vi "产品工艺设定.vi"() -> ()   [LabVIEW 2020]
panel:
  out "ALL_DEVICE":string[](array[string])
  in  "确定":bool
  in  "产品型号":u16(ring) items=[""=0, "R128"=1, "R527"=4, "R538"=5, "R92A"=3]
  in  "产品工艺":string(tree)
  in  "工位名称":i32(listbox)
  out "data":string[][](array[string])
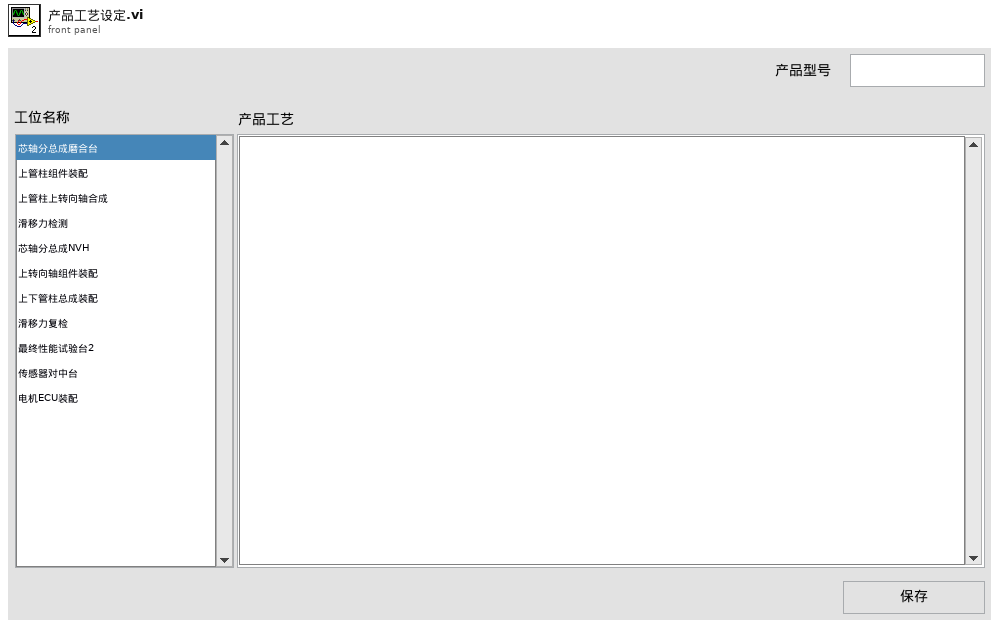
[diagram p1: front panel]
types:
  T1 = cluster{"data name":string, "drag data":variant}[]
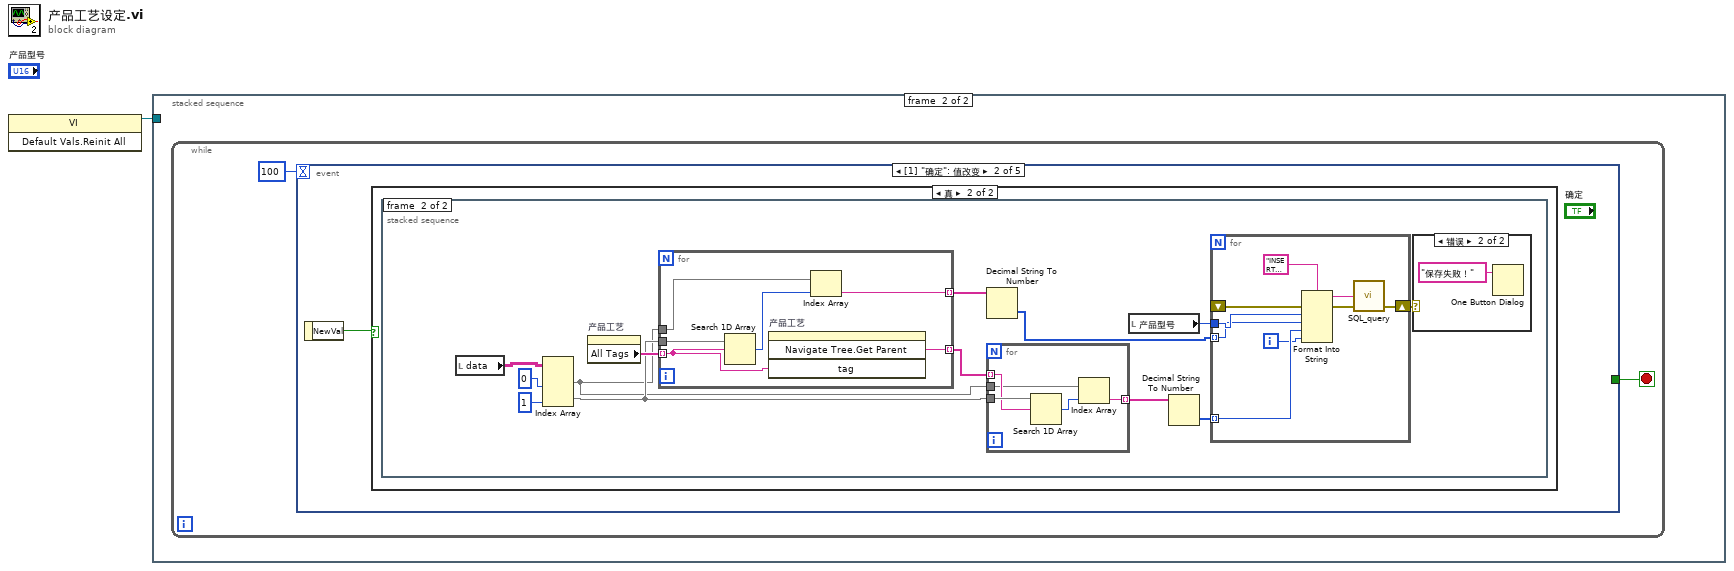
[diagram p0: block diagram]
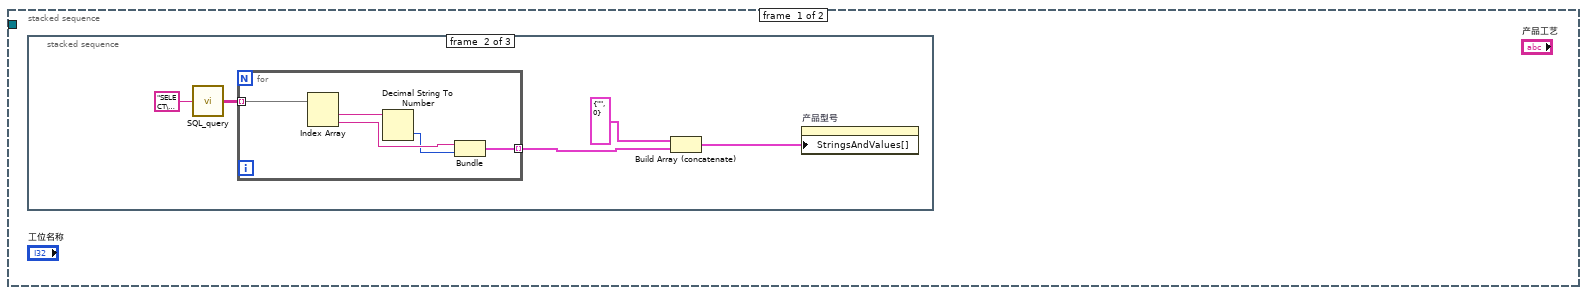
[diagram p2: hidden frame]
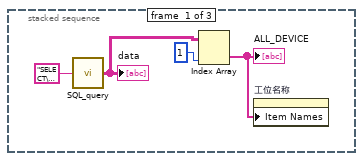
[diagram p3: hidden frame]
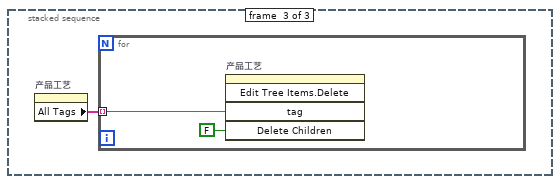
[diagram p4: hidden frame]
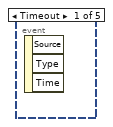
[diagram p5: hidden frame]
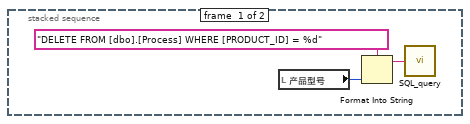
[diagram p7: hidden frame]
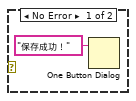
[diagram p8: hidden frame]
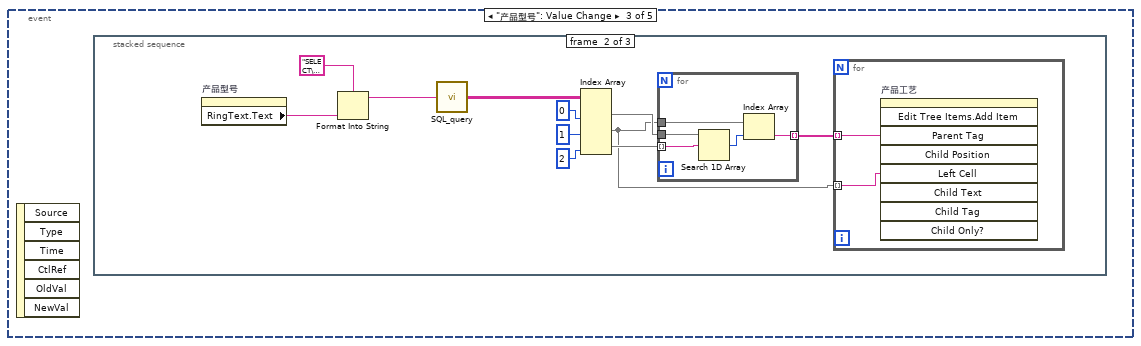
[diagram p9: hidden frame]
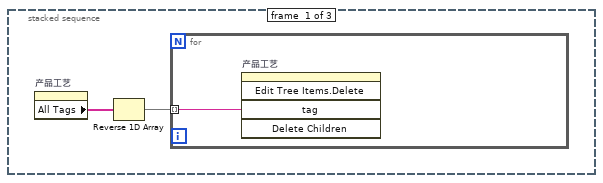
[diagram p10: hidden frame]
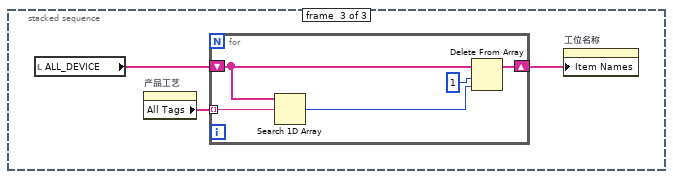
[diagram p11: hidden frame]
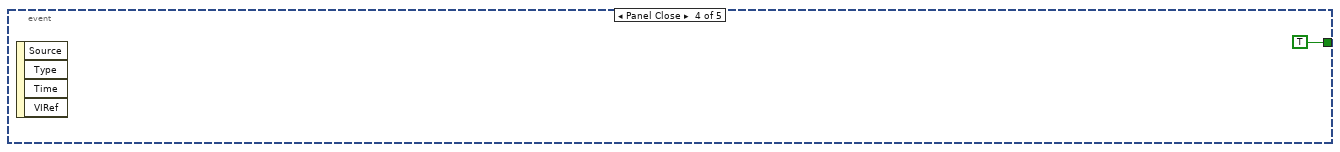
[diagram p12: hidden frame]
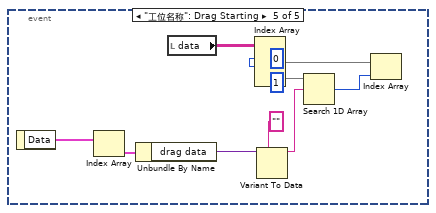
[diagram p13: hidden frame]
diagram:
  n1 = invoke class="VI" method="Default Vals.Reinit All"() -> (reference out=w1:refnum<vi>)  [unwired: 3 in, 2 out]
  n2 = stacked-sequence {
    tunnel: w1 -> [_ _]
    frame #0 {
      n3 = stacked-sequence {
        frame #0 {
          n4 = call "SQL_query.vi"("SQL query"="SELECT\ndbo.Device.DEVICE_ID,\ndbo.Device.DEVICE_NAME\n\nFROM\ndbo.Device\n") -> ("data"=w5:string[][])  [unwired: 3 in, 1 out]
          "data" <- w5
          n5 = Index Array(array=w5, index (col)=1 ("禁用的索引 (列)")) -> (element=w4:string[])  [unwired: 1 in]
          "ALL_DEVICE" <- w4
          n6 = property on="工位名称" class="LstBox (严格)"("Item Names"=w4) -> ()  [unwired: 2 in, 2 out]
        }
        frame #1 {
          n7 = call "SQL_query.vi"("SQL query"="SELECT\ndbo.Product.PRODUCT_ID,\ndbo.Product.PRODUCT_NAME\n\nFROM\ndbo.Product\n") -> ("data"=w9:string[][])  [unwired: 3 in, 1 out]
          n8 = for {
            tunnel: w9 -> [w15] mode=indexing
            tunnel: [w13] -> w10 mode=indexing
            n9 = Index Array(array=w15) -> (element #1=w12:string, element #2=w14:string)  [unwired: 2 in]
            n10 = Decimal String To Number(string=w12) -> (number=w11:i32)  [unwired: 2 in, 1 out]
            n11 = Bundle(w14, w11) -> (w13:cluster{string, i32})  [unwired: 1 in]
          }
          n12 = Build Array (concatenate)(cluster{string, i32} {"", 0}, w10) -> (w7:cluster{string, i32}[])
          n13 = property on="产品型号" class="Ring (严格)"("StringsAndValues[]"=w7) -> ()  [unwired: 2 in, 2 out]
        }
        frame #2 {
          n14 = property on="产品工艺" class="Tree (严格)"() -> ("All Tags"=w16:string[])  [unwired: 2 in, 2 out]
          n15 = for {
            tunnel: w16 -> [w18] mode=indexing
            n16 = invoke on="产品工艺" class="Tree (严格)" method="Edit Tree Items.Delete"("tag"=w18, "Delete Children"=FALSE ("删除子项？")) -> ()  [unwired: 3 in, 5 out]
          }
        }
      }
    }
    frame #1 {
      n17 = while {
        stop <- w20 stop-if-true
        n18 = event shown="[1] \"确定\": 值改变" {
          selector: _ -> [_ _ _ _ _]
          dyn-events: _ -> [_ _ _ _ _]
          timeout: 100 -> [_ _ _ _ _]
          tunnel: [_ _ _ TRUE _] -> w20
          event Timeout {
            n19 = event-data() -> ()  [unwired: 1 in, 3 out]
          }
          event "确定": Value Change {
            n20 = event-data() -> ("NewVal"=w21:bool)  [unwired: 1 in]
            n21 = case shown="真" w21 {
              frame False {
              }
              frame True {
                n22 = stacked-sequence {
                  frame #0 {
                    n23 = local read "产品型号"() -> (w23:u16)
                    n24 = Format Into String(format string="DELETE FROM [dbo].[Process] WHERE [PRODUCT_ID] = %d", w23) -> (resulting string=w22:string)  [unwired: 2 in, 1 out]
                    n25 = call "SQL_query.vi"("SQL query"=w22) -> ()  [unwired: 3 in, 2 out]
                  }
                  frame #1 {
                    n26 = local read "data"() -> (w36:string[][])
                    n27 = Index Array(array=w36, index (col) #1=0 ("禁用的索引 (列)"), index (col) #2=1 ("索引 (列)")) -> (element #1=w33:string[], element #2=w35:string[])  [unwired: 2 in]
                    n28 = property on="产品工艺" class="Tree (严格)"() -> ("All Tags"=w37:string[])  [unwired: 2 in, 2 out]
                    n29 = for {
                      tunnel: w37 -> [w57] mode=indexing
                      tunnel: [w59] -> w34 mode=indexing
                      tunnel: w33 -> [w56]
                      tunnel: w35 -> [w58]
                      tunnel: [w54] -> w29 mode=indexing
                      n30 = Search 1D Array(1D array=w58, element=w57) -> (index of element=w55:i32)  [unwired: 1 in]
                      n31 = invoke on="产品工艺" class="Tree (严格)" method="Navigate Tree.Get Parent"("tag"=w57) -> ("Navigate Tree:Get Parent"=w59:string)  [unwired: 3 in, 3 out]
                      n32 = Index Array(array=w56, index=w55) -> (element=w54:string)
                    }
                    n33 = Decimal String To Number(string=w29) -> (number=w26:i32[])  [unwired: 2 in, 1 out]
                    n34 = for {
                      tunnel: w35 -> [w52]
                      tunnel: w34 -> [w51] mode=indexing
                      tunnel: w33 -> [w50]
                      tunnel: [w49] -> w30 mode=indexing
                      n35 = Search 1D Array(1D array=w52, element=w51) -> (index of element=w53:i32)  [unwired: 1 in]
                      n36 = Index Array(array=w50, index=w53) -> (element=w49:string)
                    }
                    n37 = local read "产品型号"() -> (w28:u16)
                    n38 = Decimal String To Number(string=w30) -> (number=w27:i32[])  [unwired: 2 in, 1 out]
                    n39 = for {
                      tunnel: w27 -> [w47] mode=indexing
                      tunnel: w26 -> [w46] mode=indexing
                      tunnel: w28 -> [w48]
                      shift-right: [w42] -> w25
                      shift-left: _ -> [w41]
                      i -> [w43]
                      n40 = Format Into String(format string="INSERT INTO dbo.Process ( PRODUCT_ID, DEVICE_ID, PARENT_ID,LABVIEW_ID )\nVALUES\n\t(\n\t\t%d,\n\t\t%d,\n\t\t\t%d,\n%d)" ("格式字符串"), error in=w41, w48, w46, w47, w43) -> (resulting string=w45:string, error out=w40:errorcluster)  [unwired: 1 in]
                      n41 = call "SQL_query.vi"("error in (no error)"=w40, "SQL query"=w45) -> ("error out"=w42:errorcluster)  [unwired: 2 in, 1 out]
                    }
                    n42 = case shown="错误" w25 {
                      frame No Error {
                        n43 = One Button Dialog(message="保存成功！" ("消息")) -> ()  [unwired: 1 in, 1 out]
                      }
                      frame Error {
                        n44 = One Button Dialog(message="保存失败！" ("消息")) -> ()  [unwired: 1 in, 1 out]
                      }
                    }
                  }
                }
              }
            }
          }
          event "产品型号": Value Change {
            n45 = event-data() -> ()  [unwired: 1 in, 6 out]
            n46 = stacked-sequence {
              frame #0 {
                n47 = property on="产品工艺" class="Tree (严格)"() -> ("All Tags"=w61:string[])  [unwired: 2 in, 2 out]
                n48 = Reverse 1D Array(array=w61) -> (reversed array=w60:string[])
                n49 = for {
                  tunnel: w60 -> [w62] mode=indexing
                  n50 = invoke on="产品工艺" class="Tree (严格)" method="Edit Tree Items.Delete"("tag"=w62) -> ()  [unwired: 4 in, 5 out]
                }
              }
              frame #1 {
                n51 = property on="产品型号" class="Ring (严格)"() -> ("RingText.Text"=w67:string)  [unwired: 2 in, 2 out]
                n52 = Format Into String(format string="SELECT\ndbo.Process.DEVICE_ID,\ndbo.Device.DEVICE_NAME,\ndbo.Process.PARENT_ID\n\nFROM\ndbo.Process\nINNER JOIN dbo.Device ON dbo.Process.DEVICE_ID = dbo.Device.DEVICE_ID\nINNER JOIN dbo.Product ON dbo.Process.PRODUCT_ID = dbo.Product.PRODUCT_ID\nWHERE\ndbo.Product.PRODUCT_NAME = '%s'\nORDER BY\ndbo.Process.LABVIEW_ID ASC\n", w67) -> (resulting string=w66:string)  [unwired: 2 in, 1 out]
                n53 = call "SQL_query.vi"("SQL query"=w66) -> ("data"=w73:string[][])  [unwired: 3 in, 1 out]
                n54 = Index Array(array=w73, index (col) #1=0 ("禁用的索引 (列)"), index (col) #2=1 ("索引 (列)"), index (col) #3=2 ("索引 (列)")) -> (element #1=w68:string[], element #2=w63:string[], element #3=w69:string[])  [unwired: 3 in]
                n55 = for {
                  tunnel: w63 -> [w78]
                  tunnel: w69 -> [w79] mode=indexing
                  tunnel: w68 -> [w80]
                  tunnel: [w76] -> w64 mode=indexing
                  n56 = Search 1D Array(1D array=w80, element=w79) -> (index of element=w77:i32)  [unwired: 1 in]
                  n57 = Index Array(array=w78, index=w77) -> (element=w76:string)
                }
                n58 = for {
                  tunnel: w64 -> [w75] mode=indexing
                  tunnel: w63 -> [w74] mode=indexing
                  n59 = invoke on="产品工艺" class="Tree (严格)" method="Edit Tree Items.Add Item"("Parent Tag"=w75, "Left Cell"=w74) -> ()  [unwired: 7 in, 9 out]
                }
              }
              frame #2 {
                n60 = local read "ALL_DEVICE"() -> (w82:string[])
                n61 = property on="产品工艺" class="Tree (严格)"() -> ("All Tags"=w81:string[])  [unwired: 2 in, 2 out]
                n62 = for {
                  tunnel: w81 -> [w88] mode=indexing
                  shift-right: [w84] -> w83
                  shift-left: w82 -> [w87]
                  n63 = Search 1D Array(1D array=w87, element=w88) -> (index of element=w85:i32)  [unwired: 1 in]
                  n64 = Delete From Array(array=w87, length=1 ("长度"), index=w85) -> (array with subset deleted=w84:string[])  [unwired: 1 out]
                }
                n65 = property on="工位名称" class="LstBox (严格)"("Item Names"=w83) -> ()  [unwired: 2 in, 2 out]
              }
            }
          }
          event Panel Close {
            n66 = event-data() -> ()  [unwired: 1 in, 4 out]
          }
          event "工位名称": Drag Starting {
            n67 = event-data() -> ("Data"=w96:T1)  [unwired: 1 in]
            n68 = Index Array(array=w96) -> (element=w95:cluster{"data name":string, "drag data":variant})  [unwired: 1 in]
            n69 = Unbundle By Name(w95) -> ("drag data"=w94:variant)
            n70 = local read "data"() -> (w100:string[][])
            n71 = Index Array(array=w100, index (col) #1=0 ("禁用的索引 (列)"), index (col) #2=1 ("索引 (列)")) -> (element #1=w91:string[], element #2=w97:string[])  [unwired: 2 in]
            n72 = Variant To Data(type="", Variant=w94) -> (data=w92:string)  [unwired: 1 in, 1 out]
            n73 = Search 1D Array(1D array=w97, element=w92) -> (index of element=w90:i32)  [unwired: 1 in]
            n74 = Index Array(array=w91, index=w90) -> ()  [unwired: 1 out]
          }
        }
      }
    }
  }
